vi "actuate_currentRampExp_v0.05.vi"(0 "Phase Cluster":T4, 1 "valve Time Cluster":T3, 2 "Didn't Lift?":bool, 3 "data in":T5={"daq_ao 1"="Dev1/ao0", "daq_ai 1"="Dev1/ai0", "experiment day folder"=path "D:/DATA/8-27-15 save func testing/test.lvm", "Multiclamp init error"=0, "Multiclamp Handle Out"=0, "sampling rate (Hz)"=10000, "trial name"=""}, 5 "PhaseLetter":string, 7 "controls array in":refnum<vi>[](array[refnum]), 9 "time to wait for solution change (min)":dbl=2.5 min=0.0 step=0.01, 11 "error in":errorcluster, 12 "common cluster":T7, 13 "individual controls in":T6) -> (4 "output cluster":T1, 6 "protocol waveform":waveform(dbl)[](graph), 8 "jumptestMonitor":waveform(dbl)[](graph) caption="protocol response", 10 "control array out":refnum<vi>[](array[refnum]), 14 "experiment VI ref":refnum<vi>, 15 "error out":errorcluster)   [LabVIEW 2019]
uses:
  pipette cleaning/pressure box/cleaning_soft/controls/actuator_type.ctl
  pipette cleaning/pressure box/cleaning_soft/controls/actuator_cluster.ctl
  machine_vision/coordinate model vis/transform_properties_actuators.ctl
  machine_vision/controls/transform_cluster_actuator.ctl
  controls/NH_method.ctl
  pipette cleaning/pressure box/cleaning_soft/controls/pressure_box_type.ctl
  pipette cleaning/pressure box/cleaning_soft/controls/pressure_box_control.ctl
  multipatch/controls/multipatch_common_controls_v4.ctl
  controls/memtest_def.ctl
  multipatch/controls/multipatch_individual_controls_v5.ctl
  Controls/Data.ctl
panel:
  in  "VoltageRampValuesCluster":T2
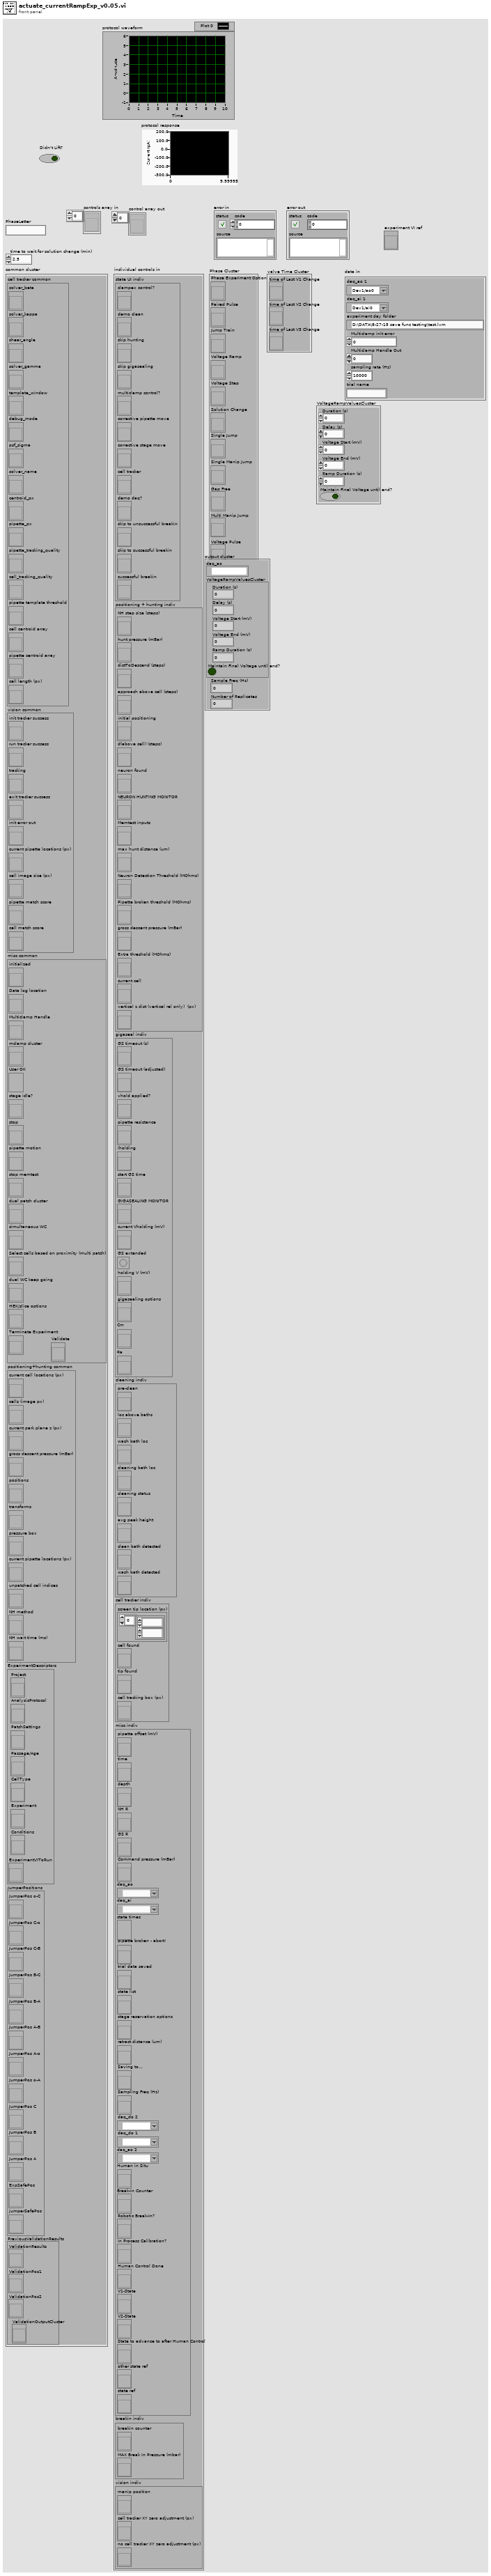
[diagram p1: front panel]
types:
  T1 = cluster{"daq_ao":tag, "VoltageRampValuesCluster":cluster{"Duration (s)":dbl, "Delay (s)":dbl, "Voltage Start (mV)":dbl, "Voltage End (mV)":dbl, "Ramp Duration (s)":dbl, "Maintain Final Voltage until end?":bool}, "Sample Freq (Hz)":dbl, "Number of Replicates":i16}
  T2 = cluster{"Duration (s)":dbl, "Delay (s)":dbl, "Voltage Start (mV)":dbl, "Voltage End (mV)":dbl, "Ramp Duration (s)":dbl, "Maintain Final Voltage until end?":bool}
  T3 = cluster{"time of Last V1 Change":refnum<vi>, "time of Last V2 Change":refnum<vi>, "time of Last V3 Change":refnum<vi>}
  T4 = cluster{"Phase Experiment Option":refnum<vi>, "Paired Pulse":refnum<vi>, "Jump Train":refnum<vi>, "Voltage Ramp":refnum<vi>, "Voltage Step":refnum<vi>, "Solution Change":refnum<vi>, "Single Jump":refnum<vi>, "Single Manip Jump":refnum<vi>, "Gap Free":refnum<vi>, "Multi Manip Jump":refnum<vi>, "Voltage Pulse":refnum<vi>, "Current Pulse":refnum<vi>, "Current Ramp":refnum<vi>, "Gap Free Iclamp":refnum<vi>}
  T5 = typedef "Data.ctl" = cluster{"daq_ao 1":tag, "daq_ai 1":tag, "experiment day folder":path, "Multiclamp init error":i32, "Multiclamp Handle Out":u32, "sampling rate (Hz)":i32, "trial name":string}
  T6 = typedef "multipatch_individual_controls_v5.ctl" = cluster{"state UI indiv":cluster{"clampex control?":refnum<vi>, "demo clean":refnum<vi>, "skip hunting":refnum<vi>, "skip gigasealing":refnum<vi>, "multiclamp control?":refnum<vi>, "corrective pipette move":refnum<vi>, "corrective stage move":refnum<vi>, "cell tracker":refnum<vi>, "demo daq?":refnum<vi>, "skip to unsuccessful breakin":refnum<vi>, "skip to successful breakin":refnum<vi>, "successful breakin":refnum<vi>}, "positioning + hunting indiv":cluster{"NH step size (steps)":refnum<vi>, "hunt pressure (mBar)":refnum<vi>, "distToDescend (steps)":refnum<vi>, "approach above cell (steps)":refnum<vi>, "initial positioning":refnum<vi>, "d(above cell) (steps)":refnum<vi>, "neuron found":refnum<vi>, "NEURON HUNTING MONITOR":refnum<vi>, "Memtest inputs":refnum<vi>, "max hunt distance (um)":refnum<vi>, "Neuron Detection Threshold (MOhms)":refnum<vi>, "Pipette broken threshold (MOhms)":refnum<vi>, "gross descent pressure (mBar)":refnum<vi>, "Extra threshold (MOhms)":refnum<vi>, "current cell":refnum<vi>, "vertical z dist (vertical rel only)  (px)":refnum<vi>}, "gigaseal indiv":cluster{"GS timeout (s)":refnum<vi>, "GS timeout (adjusted)":refnum<vi>, "vhold applied?":refnum<vi>, "pipette resistance":refnum<vi>, "Iholding":refnum<vi>, "start GS time":refnum<vi>, "GIGASEALING MONITOR":refnum<vi>, "current Vholding (mV)":refnum<vi>, "GS extended":refnum<vi>, "holding V (mV)":refnum<vi>, "gigasealing options":refnum<vi>, "Cm":refnum<vi>, "Ra ":refnum<vi>}, "cleaning indiv":cluster{"pre-clean":refnum<vi>, "loc above baths":refnum<vi>, "wash bath loc":refnum<vi>, "cleaning bath loc":refnum<vi>, "cleaning status":refnum<vi>, "avg peak height":refnum<vi>, "clean bath detected":refnum<vi>, "wash bath detected":refnum<vi>}, "cell tracker indiv":cluster{"screen tip location (px)":refnum<vi>, "cell found":refnum<vi>, "tip found":refnum<vi>, "cell tracking box (px)":refnum<vi>}, "misc indiv":cluster{"pipette offset (mV)":refnum<vi>, "time":refnum<vi>, "depth":refnum<vi>, "NH R":refnum<vi>, "GS R":refnum<vi>, "Command pressure (mBar)":refnum<vi>, "daq_ao":tag, "daq_ai":tag, "state times":refnum<vi>, "pipette broken - abort!":refnum<vi>, "trial data saved":refnum<vi>, "state list":refnum<vi>, "stage reservation options":refnum<vi>, "retract distance (um)":refnum<vi>, "Saving to...":refnum<vi>, "Sampling Freq (Hz)":refnum<vi>, "daq_do 2":tag, "daq_do 1":tag, "daq_ao 2":tag, "Human in Situ":refnum<vi>, "Break-In Counter":refnum<vi>, "Robotic Break-In?":refnum<vi>, "In Process Calibration?":refnum<vi>, "Human Control Done":refnum<vi>, "V1-State":refnum<vi>, "V2-State":refnum<vi>, "State to advance to after Human Control":refnum<vi>, "other state ref":refnum<vi>, "state ref":refnum<vi>}, "breakin indiv":cluster{"breakin counter":refnum<vi>, "MAX Break In Pressure (mbar)":refnum<vi>}, "vision indiv":cluster{"manip position":refnum<vi>, "cell tracker XY zero adjustment (px)":refnum<vi>, "no cell tracker XY zero adjustment (px)":refnum<vi>}}
  T7 = typedef "multipatch_common_controls_v4.ctl" = cluster{"cell tracker common":cluster{"solver_beta":refnum<vi>, "solver_kappa":refnum<vi>, "shear_angle":refnum<vi>, "solver_gamma":refnum<vi>, "template_window":refnum<vi>, "debug_mode":refnum<vi>, "psf_sigma":refnum<vi>, "solver_name":refnum<vi>, "centroid_px":refnum<vi>, "pipette_px":refnum<vi>, "pipette_tracking_quality":refnum<vi>, "cell_tracking_quality":refnum<vi>, "pipette template threshold":refnum<vi>, "cell centroid array":refnum<vi>, "pipette centroid array":refnum<vi>, "cell length (px)":refnum<vi>}, "vision common":cluster{"init tracker success":refnum<vi>, "run tracker success":refnum<vi>, "tracking":refnum<vi>, "exit tracker success":refnum<vi>, "init error out":refnum<vi>, "current pipette locations (px)":refnum<vi>, "cell image size (px)":refnum<vi>, "pipette match score":refnum<vi>, "cell match score":refnum<vi>}, "misc common":cluster{"initialized":refnum<vi>, "Data log location":refnum<vi>, "Multiclamp Handle":refnum<vi>, "mclamp cluster":refnum<vi>, "User OK":refnum<vi>, "stage idle?":refnum<vi>, "stop":refnum<vi>, "pipette motion":refnum<vi>, "stop memtest":refnum<vi>, "dual patch cluster":refnum<vi>, "simultaneous WC":refnum<vi>, "Select cells based on proximity (multi patch)":refnum<vi>, "dual WC keep going":refnum<vi>, "HEK/slice options":refnum<vi>, "Terminate Experiment":refnum<vi>, "Validate":refnum<vi>}, "positioning+hunting common":cluster{"current cell locations (px)":refnum<vi>, "cells (image px)":refnum<vi>, "current park plane z (px)":refnum<vi>, "gross descent pressure (mBar)":refnum<vi>, "positions":refnum<vi>, "transforms":refnum<vi>, "pressure box":refnum<vi>, "current pipette locations (px)":refnum<vi>, "unpatched cell indices":refnum<vi>, "NH method":refnum<vi>, "NH wait time (ms)":refnum<vi>}, "ExperimentDescriptors":cluster{"Project":refnum<vi>, "AnalysisProtocol":refnum<vi>, "PatchSettings":refnum<vi>, "Passage/Age":refnum<vi>, "CellType":refnum<vi>, "Experiment":refnum<vi>, "Conditions":refnum<vi>, "ExperimentVIToRun":refnum<vi>}, "JumperPositions":cluster{"JumperPos o-C":refnum<vi>, "JumperPos C-o":refnum<vi>, "JumperPos C-B":refnum<vi>, "JumperPos B-C":refnum<vi>, "JumperPos B-A":refnum<vi>, "JumperPos A-B":refnum<vi>, "JumperPos A-o":refnum<vi>, "JumperPos o-A":refnum<vi>, "JumperPos C":refnum<vi>, "JumperPos B":refnum<vi>, "JumperPos A":refnum<vi>, "ExpSafePos":refnum<vi>, "jumperSafePos":refnum<vi>}, "PreviousValidationResults":cluster{"ValidationResults":refnum<vi>, "ValidationPos1":refnum<vi>, "ValidationPos2":refnum<vi>, "ValidationOutputCluster":refnum<vi>}}
  T8 = cluster{"Which Position to use for Experiment":enum16{"Jumper Safe Position", "Experiment Safe Position", "Jumper Position A", "Jumper Position B", "Jumper Position C", "Jumper Position o-A", "Jumper Position A-o", "Jumper Position A-B", "Jumper Position B-A", "Jumper Position B-C", "Jumper Position C-B", "Jumper Position C-o", "Jumper Position o-C", "Don't Move"}, "Duration (s)":dbl, "Delay (s)":dbl, "Ramp Slope (pA/s)":dbl, "Current Start (pA)":dbl, "Replicates":dbl, "Current End (pA)":dbl, "Ramp Duration (s)":dbl, "Iholding (pA)":dbl, "Valve 1 Position":i16, "Valve 2 Position":i16, "Valve 3 Position":i16, "valve 1 used now?":bool, "valve 2 used now?":bool, "valve 3 used now? ":bool, "Maintain Final Voltage until end?":bool, "protocol Preview":waveform(dbl)[]}
  T9 = enum16{"Jumper Safe Position", "Experiment Safe Position", "Jumper Position A", "Jumper Position B", "Jumper Position C", "Jumper Position o-A", "Jumper Position A-o", "Jumper Position A-B", "Jumper Position B-A", "Jumper Position B-C", "Jumper Position C-B", "Jumper Position C-o", "Jumper Position o-C", "Don't Move"}
  T10 = enum16{"manipulator 1", "manipulator 2", "manipulator 3", "manipulator 4"}
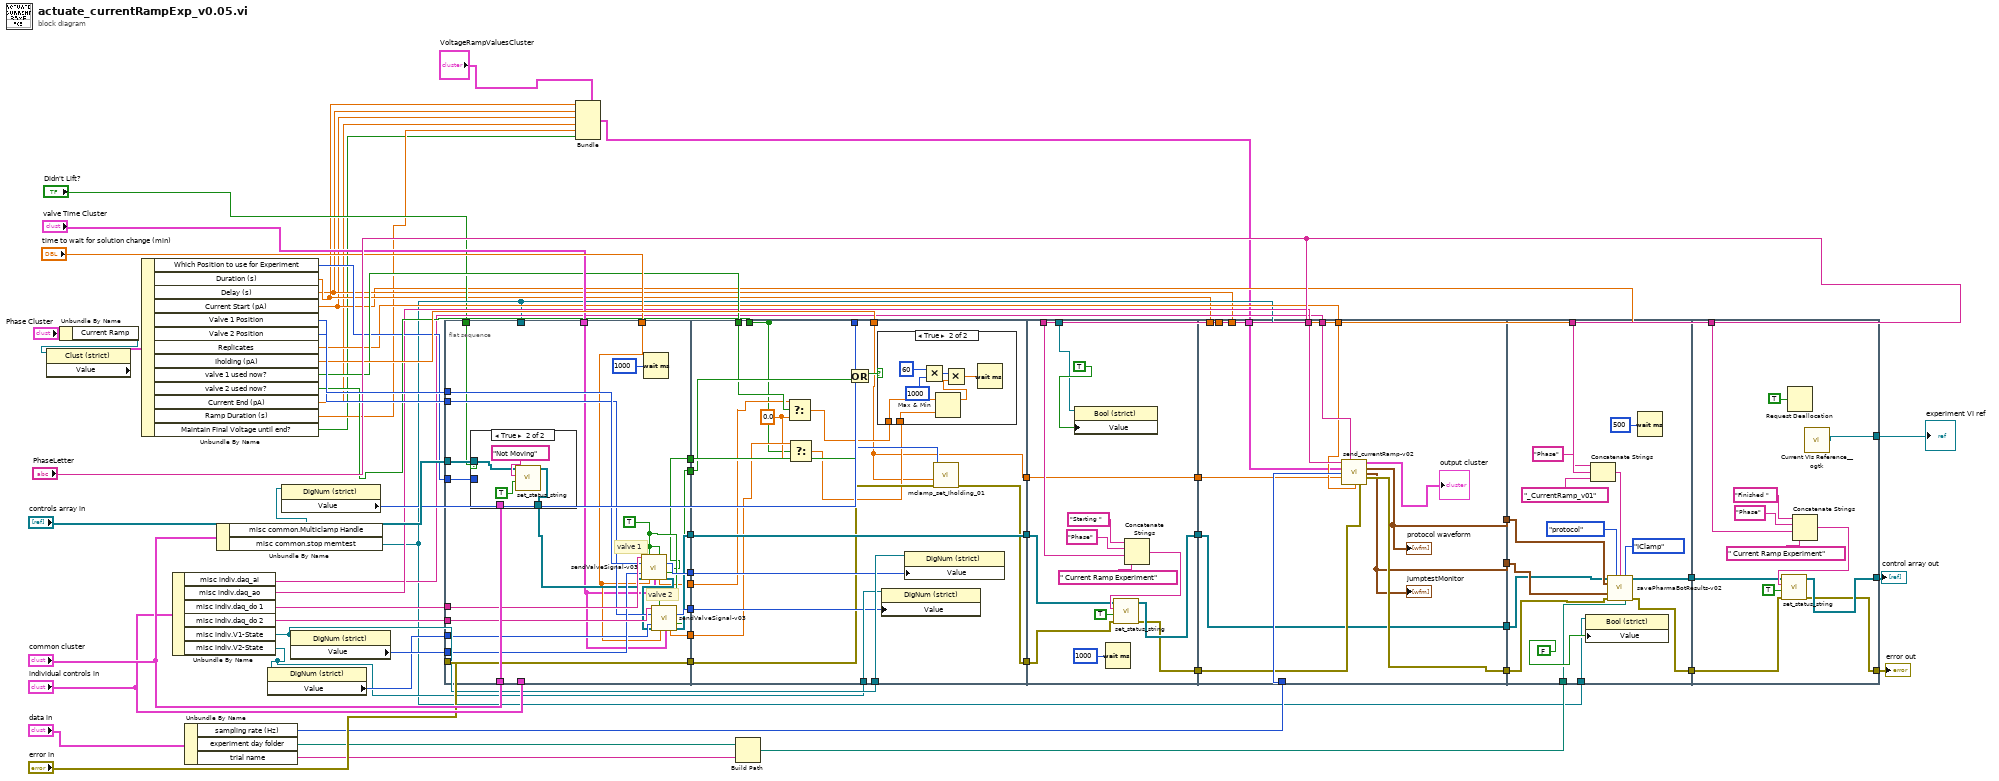
[diagram p0: block diagram]
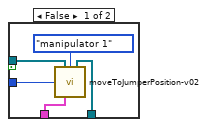
[diagram p2: hidden frame]
diagram:
  n1 = Unbundle By Name("Phase Cluster") -> ("Current Ramp"=w43:refnum<vi>)
  n2 = property class="Clust (strict)"(reference=w43) -> ("Value"=w42:T8)  [unwired: 1 in, 2 out]
  n3 = Unbundle By Name(w42) -> ("Which Position to use for Experiment"=w18:T9, "Duration (s)"=w11:dbl, "Delay (s)"=w10:dbl, "Current Start (pA)"=w9:dbl, "Valve 1 Position"=w41:i16, "Valve 2 Position"=w40:i16, "Replicates"=w17:dbl, "Iholding (pA)"=w27:dbl, "valve 1 used now?"=w20:bool, "valve 2 used now?"=w19:bool, "Current End (pA)"=w8:dbl, "Ramp Duration (s)"=w7:dbl, "Maintain Final Voltage until end?"=w3:bool)
  n4 = Unbundle By Name("individual controls in") -> ("misc indiv.daq_ai"=w14:tag, "misc indiv.daq_ao"=w15:tag, "misc indiv.daq_do 1"=w63:tag, "misc indiv.daq_do 2"=w62:tag, "misc indiv.V1-State"=w54:refnum<vi>, "misc indiv.V2-State"=w53:refnum<vi>)
  n5 = Unbundle By Name("data in") -> ("sampling rate (Hz)"=w16:i32, "experiment day folder"=w47:path, "trial name"=w46:string)
  n6 = Unbundle By Name("common cluster") -> ("misc common.Multiclamp Handle"=w26:refnum<vi>, "misc common.stop memtest"=w13:refnum<vi>)
  n7 = property class="DigNum (strict)"(reference=w53) -> ("Value"=w55:u16)  [unwired: 1 in, 2 out]
  n8 = property class="DigNum (strict)"(reference=w26) -> ("Value"=w25:u32)  [unwired: 1 in, 2 out]
  n9 = property class="DigNum (strict)"(reference=w54) -> ("Value"=w56:u16)  [unwired: 1 in, 2 out]
  n10 = flat-sequence {
    tunnel: "common cluster" -> [w88]
    tunnel: "individual controls in" -> [_]
    tunnel: [w85] -> w58
    tunnel: [w82] -> w52
    tunnel: [w81] -> w51
    tunnel: [w75] -> w34
    tunnel: [w73] -> w29
    tunnel: [w72] -> w28
    tunnel: "time to wait for solution change (min)" -> [w71]
    tunnel: "valve Time Cluster" -> [w70]
    tunnel: [w69] -> w22
    tunnel: [w68] -> w21
    tunnel: w13 -> [_]
    tunnel: "Didn't Lift?" -> [w66]
    tunnel: w18 -> [w89]
    tunnel: w63 -> [w87]
    tunnel: w62 -> [w86]
    tunnel: "error in" -> [w85]
    tunnel: w56 -> [w84]
    tunnel: w55 -> [w83]
    tunnel: w41 -> [w80]
    tunnel: w40 -> [w79]
    tunnel: "controls array in" -> [w78]
    tunnel: [w107] -> w59
    tunnel: w58 -> [w109]
    tunnel: w54 -> [w117]
    tunnel: w53 -> [w116]
    tunnel: w52 -> [w115]
    tunnel: w51 -> [w114]
    tunnel: [w113] -> w35
    tunnel: w34 -> [w113]
    tunnel: w29 -> [w111]
    tunnel: w28 -> [w110]
    tunnel: w27 -> [w99]
    tunnel: w25 -> [w108]
    tunnel: w22 -> [w104]
    tunnel: w21 -> [w103]
    tunnel: w20 -> [w105]
    tunnel: [w100] -> _
    tunnel: w19 -> [w100]
    tunnel: [w99] -> w4
    tunnel: w13 -> [w126]
    tunnel: [w128] -> w60
    tunnel: w59 -> [w129]
    tunnel: [w130] -> w36
    tunnel: w35 -> [w131]
    tunnel: "PhaseLetter" -> [w132]
    tunnel: [w125] -> w5
    tunnel: w4 -> [w125]
    tunnel: w14 -> [w150]
    tunnel: w15 -> [w149]
    tunnel: w60 -> [w144]
    tunnel: [w147] -> w50
    tunnel: [w141] -> w49
    tunnel: w17 -> [w145]
    tunnel: w11 -> [_]
    tunnel: w16 -> [w146]
    tunnel: w9 -> [_]
    tunnel: w10 -> [_]
    tunnel: [w143] -> w39
    tunnel: [w142] -> w37
    tunnel: w36 -> [w142]
    tunnel: w6 -> [w140]
    tunnel: w5 -> [w139]
    tunnel: w13 -> [w165]
    tunnel: w50 -> [w164]
    tunnel: w49 -> [w163]
    tunnel: w45 -> [w160]
    tunnel: "PhaseLetter" -> [w158]
    tunnel: w39 -> [w155]
    tunnel: w37 -> [w154]
    tunnel: [w152] -> w32
    tunnel: [w153] -> w31
    tunnel: [w172] -> w33
    tunnel: [w171] -> w57
    tunnel: w32 -> [w170]
    tunnel: w31 -> [w173]
    tunnel: "PhaseLetter" -> [w169]
    tunnel: [w168] -> w1
    frame #0 {
      w74 = TRUE ("Set Status")
      # "valve 2"
      # "valve 1"
      n11 = case shown="True" w66 {
        tunnel: w89 -> [w94 _]
        tunnel: w88 -> [w93 _]
        tunnel: w78 -> [w91 w95]
        tunnel: [w90 w96] -> w77
        frame False {
          n12 = call "moveToJumperPosition-v02.vi"("which manipulator"=T10."manipulator 1", "controls array in"=w91, "Which Jumper Position to move to?"=w94, "common cluster"=w93) -> ("control array out"=w90:refnum<vi>[])  [unwired: 10 in, 1 out]
        }
        frame True {
          n13 = call "set_status_string.vi"("new line?"=TRUE, "status string in"="Not Moving", "controls array"=w95) -> ("controls array out"=w96:refnum<vi>[])  [unwired: 7 in, 1 out]
        }
      }
      n14 = call "sendValveSignal-v03.vi"("daq_do"=w87, "Set Status"=w74, "Valve1?"=w74, "ChangeToValve"=w80, "CurrentValve"=w84, "controls array in"=w77, "time to wait for solution change (min)"=w71, "valve Time Cluster"=w70) -> ("ValveSetTo"=w81:u16, "valve changed?"=w73:bool, "additional time to wait (min)"=w69:dbl, "control array out"=w76:refnum<vi>[])  [unwired: 4 in]
      n15 = Wait (ms)(milliseconds to wait=u32 1000) -> ()  [unwired: 1 out]
      n16 = call "sendValveSignal-v03.vi"("daq_do"=w86, "Set Status"=w74, "ChangeToValve"=w79, "CurrentValve"=w83, "controls array in"=w76, "time to wait for solution change (min)"=w71, "valve Time Cluster"=w70) -> ("ValveSetTo"=w82:u16, "valve changed?"=w72:bool, "additional time to wait (min)"=w68:dbl, "control array out"=w75:refnum<vi>[])  [unwired: 5 in]
    }
    frame #1 {
      w101 = 0.0 ("f")
      n17 = Select(t=w104, s=w105, f=w101) -> (s? t:f=w106:dbl)
      n18 = Select(t=w103, s=w100, f=w101) -> (s? t:f=w102:dbl)
      n19 = Or(x=w111, y=w110) -> (x .or. y?=w112:bool)
      n20 = case shown="True" w112 {
        tunnel: w106 -> [_ w120]
        tunnel: w102 -> [_ w119]
        frame False {
        }
        frame True {
          n21 = Multiply(x=u32 60 ("milliseconds to wait"), y=u32 1000) -> (x*y=w122:u32)
          n22 = Max & Min(x=w120, y=w119) -> (max(x,y)=w118:dbl)  [unwired: 1 out]
          n23 = Multiply(x=w122, y=w118) -> (x*y=w121:dbl)
          n24 = Wait (ms)(milliseconds to wait=w121) -> ()  [unwired: 1 out]
        }
      }
      n25 = property class="DigNum (strict)"(reference=w116, "Value"=w115) -> ()  [unwired: 1 in, 2 out]
      n26 = property class="DigNum (strict)"(reference=w117, "Value"=w114) -> ()  [unwired: 1 in, 2 out]
      n27 = call "mclamp_set_Iholding_01.vi"("error in (no error)"=w109, "set holding (pA)"=w99, "Multiclamp Handle Out"=w108) -> ("error out"=w107:errorcluster)  [unwired: 7 in, 1 out]
    }
    frame #2 {
      n28 = property class="Bool (strict)"(reference=w126, "Value"=TRUE ("stop memtest")) -> ()  [unwired: 1 in, 2 out]
      n29 = Wait (ms)(milliseconds to wait=u32 1000) -> ()  [unwired: 1 out]
      n30 = Concatenate Strings("Starting " ("string"), "Phase" ("string"), w132, " Current Ramp Experiment" ("string")) -> (w134:string)
      n31 = call "set_status_string.vi"("error in"=w129, "new line?"=TRUE, "status string in"=w134, "controls array"=w131) -> ("error out"=w128:errorcluster, "controls array out"=w130:refnum<vi>[])  [unwired: 6 in]
    }
    frame #3 {
      n32 = call "send_currentRamp-v02.vi"("daq_ao"=w149, "daq_ai"=w150, "VoltageRampValuesCluster"=w140, "Sample Freq (Hz)"=w146, "set holding (mV)"=w139, "Number of Replicates"=w145, "error in"=w144) -> ("output cluster"=→"output cluster":T1, "output waveform"=w147:waveform(dbl)[], "protocol response"=w141:waveform(dbl)[], "error out"=w143:errorcluster)  [unwired: 5 in]
      "jumptestMonitor" <- w141
      "protocol waveform" <- w147
    }
    frame #4 {
      n33 = property class="Bool (strict)"(reference=w165, "Value"=FALSE ("stop memtest")) -> ()  [unwired: 1 in, 2 out]
      n34 = Concatenate Strings("Phase" ("string"), w158, "_CurrentRamp_v01" ("string")) -> (w159:string)
      n35 = call "savePharmaBotResults-v02.vi"("controls array"=w154, "protocol or memtest"=enum16{"protocol", "memtest", "validation"}."protocol", "ExpPhase"=w159, "which clamp"=enum16{"VClamp", "IClamp"}."IClamp", "protocol waveform"=w164, "protocol response"=w163, "error in"=w155, "Save to (folder dir)"=w160) -> ("controls array out"=w153:refnum<vi>[], "error out"=w152:errorcluster)  [unwired: 6 in]
      n36 = Wait (ms)(milliseconds to wait=u32 500) -> ()  [unwired: 1 out]
    }
    frame #5 {
      n37 = Request Deallocation(TRUE ("flag")) -> ()
      n38 = Concatenate Strings("Finished " ("string"), "Phase" ("string"), w169, " Current Ramp Experiment" ("string")) -> (w175:string)
      n39 = call "set_status_string.vi"("error in"=w170, "new line?"=TRUE, "status string in"=w175, "controls array"=w173) -> ("error out"=w171:errorcluster, "controls array out"=w172:refnum<vi>[])  [unwired: 6 in]
      n40 = call "Current VIs Reference__ogtk.vi"() -> ("Current VI's reference"=w168:refnum<vi>)  [unwired: 5 in]
    }
  }
  n41 = Bundle(cluster="VoltageRampValuesCluster", "Duration (s)"=w11, "Delay (s)"=w10, "Voltage Start (mV)"=w9, "Voltage End (mV)"=w8, "Ramp Duration (s)"=w7, "Maintain Final Voltage until end?"=w3) -> (w6:T2)
  n42 = Build Path(base path=w47, name or relative path=w46) -> (appended path=w45:path)
  "error out" <- w57
  "control array out" <- w33
  "experiment VI ref" <- w1
